vi "DumbDash Find Control Names.vi"(11 "Controls":refnum<vi>[](array[refnum])) -> (3 "Dashboard Names":string[](array[string]))   [LabVIEW 2014]
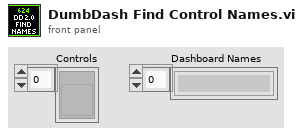
[diagram p1: front panel]
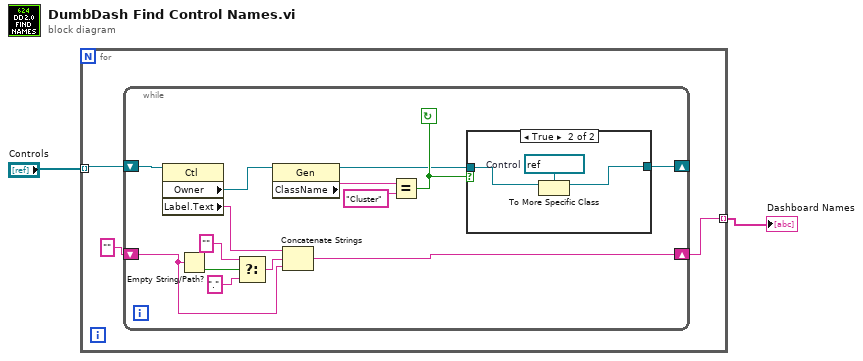
[diagram p0: block diagram]
diagram:
  n1 = for {
    tunnel: "Controls" -> [w4] mode=indexing
    tunnel: [w5] -> w2 mode=indexing
    n2 = while {
      shift-right: [w6] -> _
      shift-left: w4 -> [w16]
      shift-right: [w14] -> w5
      shift-left: "" ("Label.Text") -> [w9]
      stop <- w8 continue-if-true
      n3 = property class="Ctl"(reference=w16) -> ("Owner"=w19:refnum<vi>, "Label.Text"=w15:string)  [unwired: 1 in, 2 out]
      n4 = Empty String/Path?(string/path=w9) -> (empty?=w13:bool)
      n5 = Select(t="" ("Label.Text"), s=w13, f=".") -> (s? t:f=w10:string)
      n6 = property class="Gen"(reference=w19) -> (reference out=w7:refnum<vi>, "ClassName"=w18:string)  [unwired: 1 in, 1 out]
      n7 = Concatenate Strings(w15, w10, w9) -> (w14:string)
      n8 = Equal?(x=w18, y="Cluster") -> (x = y?=w8:bool)
      n9 = case shown="True" w8 {
        tunnel: w7 -> [_ w21]
        tunnel: [_ w20] -> w6
        frame False {
        }
        frame True {
          w22 = refnum<vi> refnum  # Control
          n10 = To More Specific Class(target class=w22, reference=w21) -> (specific class reference=w20:refnum<vi>)  [unwired: 1 in, 1 out]
        }
      }
    }
  }
  "Dashboard Names" <- w2
